vi "Extract Config.vi"(2 "Config":u8[](array[numeric])) -> (5 "OS":bool, 6 "Config Bits":bool[](array[boolean]), 7 "MUX":T1(ring), 8 "MODE":bool, 9 "PGA":T2(ring), 10 "DR":T3(ring))   [LabVIEW 2021]
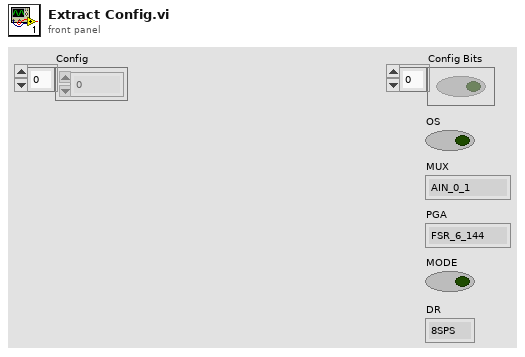
[diagram p1: front panel]
types:
  T1 = enum16{"AIN_0_1", "AIN_0_3", "AIN_1_3", "AIN_2_3", "AIN_0_G", "AIN_1_G", "AIN_2_G", "AIN_3_G"}
  T2 = enum16{"FSR_6_144", "FSR_4_096", "FSR_2_048", "FSR_1_024", "FSR_0_512", "FSR_0_256"}
  T3 = enum16{"8SPS", "16SPS", "32SPS", "64SPS", "128SPS", "250SPS", "475SPS", "860SPS"}
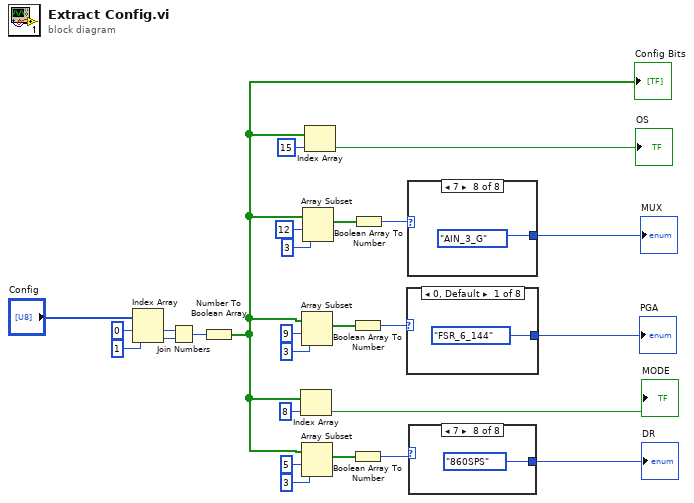
[diagram p0: block diagram]
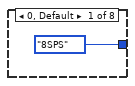
[diagram p2: hidden frame]
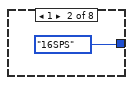
[diagram p3: hidden frame]
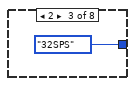
[diagram p4: hidden frame]
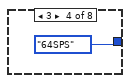
[diagram p5: hidden frame]
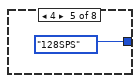
[diagram p6: hidden frame]
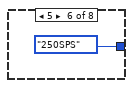
[diagram p7: hidden frame]
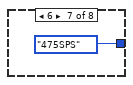
[diagram p8: hidden frame]
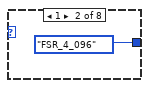
[diagram p9: hidden frame]
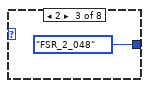
[diagram p10: hidden frame]
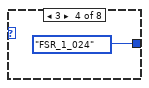
[diagram p11: hidden frame]
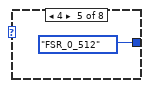
[diagram p12: hidden frame]
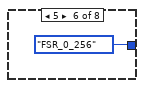
[diagram p13: hidden frame]
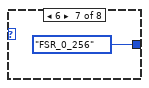
[diagram p14: hidden frame]
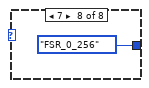
[diagram p15: hidden frame]
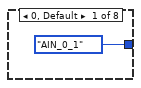
[diagram p16: hidden frame]
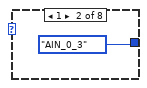
[diagram p17: hidden frame]
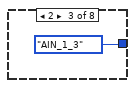
[diagram p18: hidden frame]
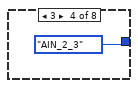
[diagram p19: hidden frame]
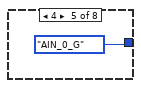
[diagram p20: hidden frame]
diagram:
  n1 = Index Array(array="Config", index #1=0 ("index"), index #2=1 ("index")) -> (element #1=w5:u8, element #2=w4:u8)
  n2 = Join Numbers(hi=w5, lo=w4) -> ((hi.lo)=w6:u16)
  n3 = Number To Boolean Array(number=w6) -> (Boolean array=w24:bool[])
  "Config Bits" <- w24
  n4 = Index Array(array=w24, index=8) -> (element=→"MODE":bool)
  n5 = Array Subset(array=w24, index=9, length=3) -> (w16:bool[])
  n6 = Array Subset(array=w24, index=5, length=3) -> (w23:bool[])
  n7 = Array Subset(array=w24, index=12, length=3) -> (w11:bool[])
  n8 = Index Array(array=w24, index=15) -> (element=→"OS":bool)
  n9 = Boolean Array To Number(Boolean array=w16) -> (number=w17:u32)
  n10 = Boolean Array To Number(Boolean array=w23) -> (number=w25:u32)
  n11 = Boolean Array To Number(Boolean array=w11) -> (number=w12:u32)
  n12 = case shown="0, Default" w17 {
    tunnel: [T2."FSR_6_144" T2."FSR_4_096" T2."FSR_2_048" T2."FSR_1_024" T2."FSR_0_512" T2."FSR_0_256" T2."FSR_0_256" T2."FSR_0_256"] -> w18
    frame 0, Default {
    }
    frame 1 {
    }
    frame 2 {
    }
    frame 3 {
    }
    frame 4 {
    }
    frame 5 {
    }
    frame 6 {
    }
    frame 7 {
    }
  }
  "PGA" <- w18
  n13 = case shown="7" w12 {
    tunnel: [T1."AIN_0_1" T1."AIN_0_3" T1."AIN_1_3" T1."AIN_2_3" T1."AIN_0_G" T1."AIN_1_G" T1."AIN_2_G" T1."AIN_3_G"] -> w13
    frame 0, Default {
    }
    frame 1 {
    }
    frame 2 {
    }
    frame 3 {
    }
    frame 4 {
    }
    frame 5 {
    }
    frame 6 {
    }
    frame 7 {
    }
  }
  "MUX" <- w13
  n14 = case shown="7" w25 {
    tunnel: [T3."8SPS" T3."16SPS" T3."32SPS" T3."64SPS" T3."128SPS" T3."250SPS" T3."475SPS" T3."860SPS"] -> w26
    frame 0, Default {
    }
    frame 1 {
    }
    frame 2 {
    }
    frame 3 {
    }
    frame 4 {
    }
    frame 5 {
    }
    frame 6 {
    }
    frame 7 {
    }
  }
  "DR" <- w26
